vi "Write Flow Control.vi"(8 "error in (no error)":errorcluster, 10 "flow control":u16(ring) items=["None", "XON/XOFF", "RTS/CTS", "XON/XOFF & RTS/CTS", "DTR/DSR", "XON/XOFF & DTR/DSR"], 11 "serial master in":refnum<class "Serial Master.lvclass">) -> (0 "error out":errorcluster, 3 "serial master out":refnum<class "Serial Master.lvclass">)   [LabVIEW 2018, in "SubVIs.lvlib" / "Serial Master.lvclass"]
uses:
  Serial Master.lvclass
  Serial Master.lvclass/Serial Master.ctl
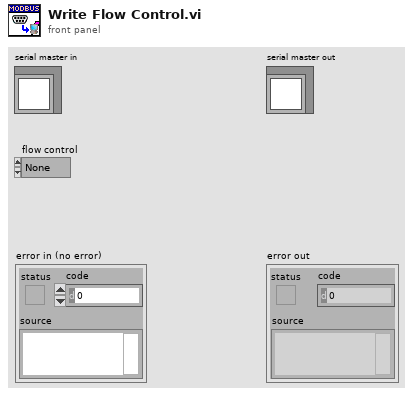
[diagram p1: front panel]
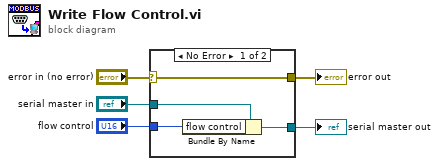
[diagram p0: block diagram]
diagram:
  n1 = case shown="No Error" "error in (no error)" {
    selector: "error in (no error)" -> [w9 w10]
    tunnel: [w9 w10] -> w4
    tunnel: [w7 w11] -> w2
    tunnel: "serial master in" -> [w8 w11]
    tunnel: "flow control" -> [w6 _]
    frame No Error {
      n2 = Bundle By Name(cluster=w8, "flow control"=w6) -> (w7:refnum<class "Serial Master.lvclass">)
    }
    frame Error {
    }
  }
  "error out" <- w4
  "serial master out" <- w2
